vi "Set Configuration.vi"(8 "error in (no error)":errorcluster, 10 "configuration":refnum<class "Configuration.lvclass">, 11 "User Interface in":refnum<class "User Interface.lvclass">) -> (0 "error out":errorcluster, 3 "User Interface out":refnum<class "User Interface.lvclass">)   [LabVIEW 2019, in "DSF Core.lvlib" / "User Interface.lvclass"]
uses:
  User Interface.lvclass
  Configuration/Configuration.lvclass
  User Interface.lvclass/User Interface.ctl
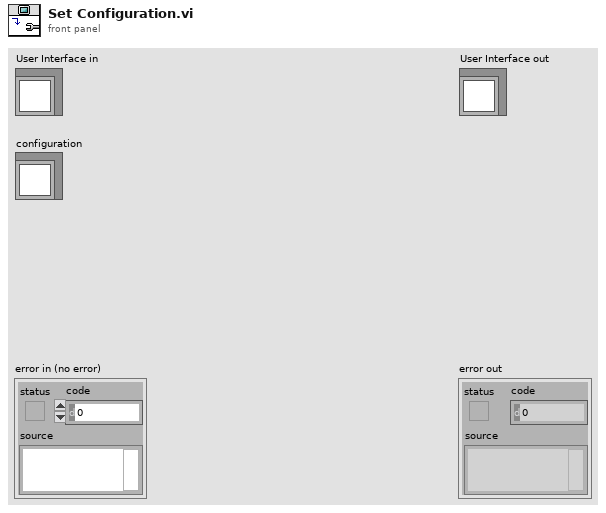
[diagram p1: front panel]
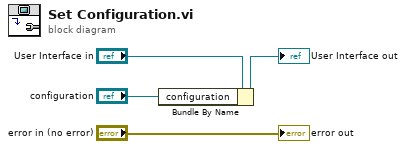
[diagram p0: block diagram]
diagram:
  n1 = Bundle By Name(cluster="User Interface in", "configuration"="configuration") -> (→"User Interface out":refnum<class "User Interface.lvclass">)
  "error out" <- "error in (no error)"
